vi "Pulsed BPSK Modulator - Channel 0.vi"() -> ()   [LabVIEW 2023]
uses:
  <vilib>/rvi/interface/nirviMethod/nirviMethod.xnode
  <vilib>/rvi/interface/nirviCloseFPGA/nirviCloseFPGA.xnode
  <vilib>/rvi/interface/nirviReadWriteControl/nirviReadWriteControl.xnode
  <vilib>/rvi/errors/niLvFpgaMergeErrorWithErrorCode.vi
  <vilib>/rvi/interface/Simulation/niFpgaSimulationCallBeginRW.vi
  <vilib>/rvi/errors/niLvFpgaAdjustHostInterfaceError.vi
  Support/Pulsed BPSK Host Support.lvlib
  <vilib>/addons/Modulation/niDMT.lvlib
  Shared/AWGN/AWGN.lvlib
  <vilib>/FPGAPlugInAG/Dynamic/niLvFpga_ReadFifo_Dynamic.vi
  <vilib>/addons/Modulation/Analog/controls/Complex Data Waveform.ctl
  <vilib>/addons/Modulation/niAMT.lvlib
  Shared/BER/Host/BER Host.lvclass
  Shared/FIR/FIR.lvlib
  Support/Public/FPGA Refnum.ctl
  Shared/AWGN/typedefs/Output Type Selection.ctl
  <vilib>/DLsc/v1/Host/Link Engine/DLsc Link Engine v1 Host.lvlib
  <vilib>/FPGAPlugInAG/Dynamic/niLvFpga_Close_Dynamic.vi
  2aa000c3-8f04-4506-bfc8-0c9442f73a61.vi
  5cab5cb4-fad3-4148-b0d2-6afb77881806.vi
  27528e13-72c1-4a4e-be7c-d3d202733046.vi
  35aca2bc-a3d1-4f8c-b8ac-3d3d75dd1f08.vi
  <vilib>/DLsc/v1/Host/Protocols/Aurora 64b66b/Extension/Aurora 64b66b Extension.lvlib
  <vilib>/DLsc/v1/Host/Link Engine/Disable Links - Single.vi
  <vilib>/addons/Modulation/Digital/General/MT Apply Matched Filter (Generic).vi
  <vilib>/addons/Modulation/Digital/General/MT Align to Ideal Symbols (Generic).vi
  <vilib>/Utility/error.llb/Error Cluster From Error Code.vi
  NiFpgaLv.dll
  <vilib>/DLsc/v1/Host/Link Engine/Enable Links - Single.vi
  <vilib>/DLsc/v1/Host/Link Engine/Commit Links - Single.vi
  <vilib>/DLsc/v1/Host/Protocols/Aurora 64b66b/Extension/Configure TX - Single.vi
  <vilib>/DLsc/v1/Host/Link Engine/Add Hardware - Single.vi
  <vilib>/FPGAPlugInAG/Dynamic/niLvFpga_Download_Dynamic.vi
  <vilib>/FPGAPlugInAG/Dynamic/niLvFpga_Run_Dynamic.vi
  <vilib>/DLsc/v1/Host/Link Engine/Close References - Single.vi
  <vilib>/FPGAPlugInAG/Dynamic/niLvFpga_ConfigureFifo_Dynamic.vi
  <vilib>/FPGAPlugInAG/Dynamic/niLvFpga_StartFifo_Dynamic.vi
  <vilib>/FPGAPlugInAG/Dynamic/niLvFpga_WriteFifo_Dynamic.vi
  <vilib>/userDefined/High Color/nirio_resource_hc.ctl
  Shared/BER/FPGA/PRBS/PRBS Degree Selection.ctl
  Shared/BER/FPGA/PRBS/PRBS.lvlib
panel:
  in  "disable DL":bool
  in  "enable DL":bool
  in  "Signal Parameters.0":T2={"Symbol Rate (Hz)"=400000000.0, "Pulse Parameters"={"Payload Length"=800, "Off Symbol Length"=800, "Preamble Symbol"=449838109, "PN Order"=4}} {"Pulse Parameters"."PN Order" items=["7", "9", "10", "11", "15", "17", "18", "20", "21", "22", "23", "25"]; "Pulse Parameters"."Preamble Symbol" format="%.0x"; "Symbol Rate (Hz)" format="%#_6p"}
  in  "Eb/N0 (dB).0":dbl=30.0 min=0.0 max=100.0 step=1.0 format="%.2g"
  in  "Power Scaling.0":dbl=1.0 min=0.0 max=1.0 step=0.002 format="%_5g"
  in  "Generation Mode.0":string(combo)="Pulsed BPSK Modulator"
  in  "Sweeping Type.0":enum16{"Eb/N0", "Power"}(ring)
  in  "Run Sweep":bool
  out "IQ Constellation":T3(graph)
  out "Bitfile Redownloaded":bool
  in  "Coprocessor Bitfile Path":path=path "C:/Users/ADG-RF/Desktop/Modems/pulsed_bpsk_modem_dmsc_7903_00_x420_single.lvbitx"
  in  "Coprocessor Device Name":T4="7903"
  in  "stop":bool
  out "Status":string
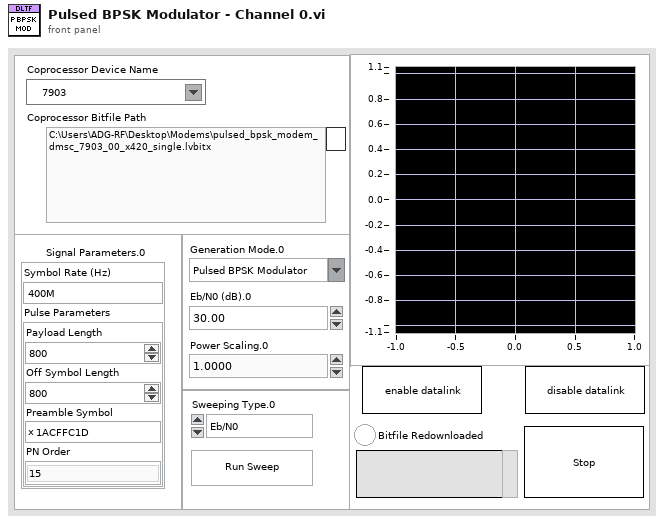
[diagram p1: front panel]
types:
  T1 = typedef "Modems Shared.lvlib/PRBS.lvlib/PRBS Degree Selection.ctl" = u16
  T2 = cluster{"Symbol Rate (Hz)":dbl, "Pulse Parameters":cluster{"Payload Length":u16, "Off Symbol Length":u16, "Preamble Symbol":i32, "PN Order":T1}}
  T3 = cluster{"constellation":dbl[], "oversampled data":dbl[]}[]
  T4 = typedef "nirio_resource_hc.ctl" = tag
  T5 = cluster{"dstepid":u16, "nummdata":fxp<+,5,5>, "pkttype":fxp<+,3,3>, "burst length":u16, "vector length":u16, "vc":fxp<+,6,6>}
  T6 = typedef "Pulsed BPSK Host Support.lvlib/FPGA Refnum.ctl" = refnum<k20>
  T7 = typedef "DLsc Link Engine v1 Host.lvlib/DLsc Session.lvclass/Session Handle.ctl" = refnum<data-value>
  T8 = typedef "DLsc Link Engine v1 Host.lvlib/DLsc Session.lvclass/Device Address Information.ctl" = cluster{"device name":string, "bitfile path":path}
  T9 = cluster{"On Symbol Count":u16, "Off Symbol Count":u16, "filter length":u16, "Preamble Count":u16}
  T10 = cluster{"AWGN Seed":fxp<+,25,25>, "AWGN scaling":fxp<+,16,0>, "output type selection":i16, "power scaling":fxp<+,16,0>}
  T11 = cluster{"filter select":enum8{"None", "I Inline", "I Cross", "Q Cross", "Q Inline"}, "coef load":bool, "coef write":bool, "coef data":fxp<+/-,18,1>}
  T12 = typedef "Modems Shared.lvlib/AWGN.lvlib/Output Type Selection.ctl" = enum16{"I16.1", "I16.2", "I16.3", "I16.4", "I16.5", "AWGN"}
  T13 = enum16{"FSK", "PSK", "QAM", "MSK", "PAM", "ASK", "CPM"}
  T14 = enum16{"none", "Raised Cosine", "Root Raised Cos", "Gaussian"}
  T15 = typedef "niAMT.lvlib/Complex Data Waveform.ctl" = cluster{"t0":dbl, "dt":dbl, "Y":cdb[]}
  T16 = cluster{"Inc":bool, "Sweeping Type":enum16{"Eb/N0", "Power"}, "Sweeping Start Point":cluster{"Eb/N0":dbl, "Power Scaling":dbl}, "Sweeping Current Point":cluster{"Eb/N0":dbl, "Power Scaling":dbl}}
  T17 = cluster{"Eb/N0 (dB).0":dbl, "Power Scaling.0":dbl}
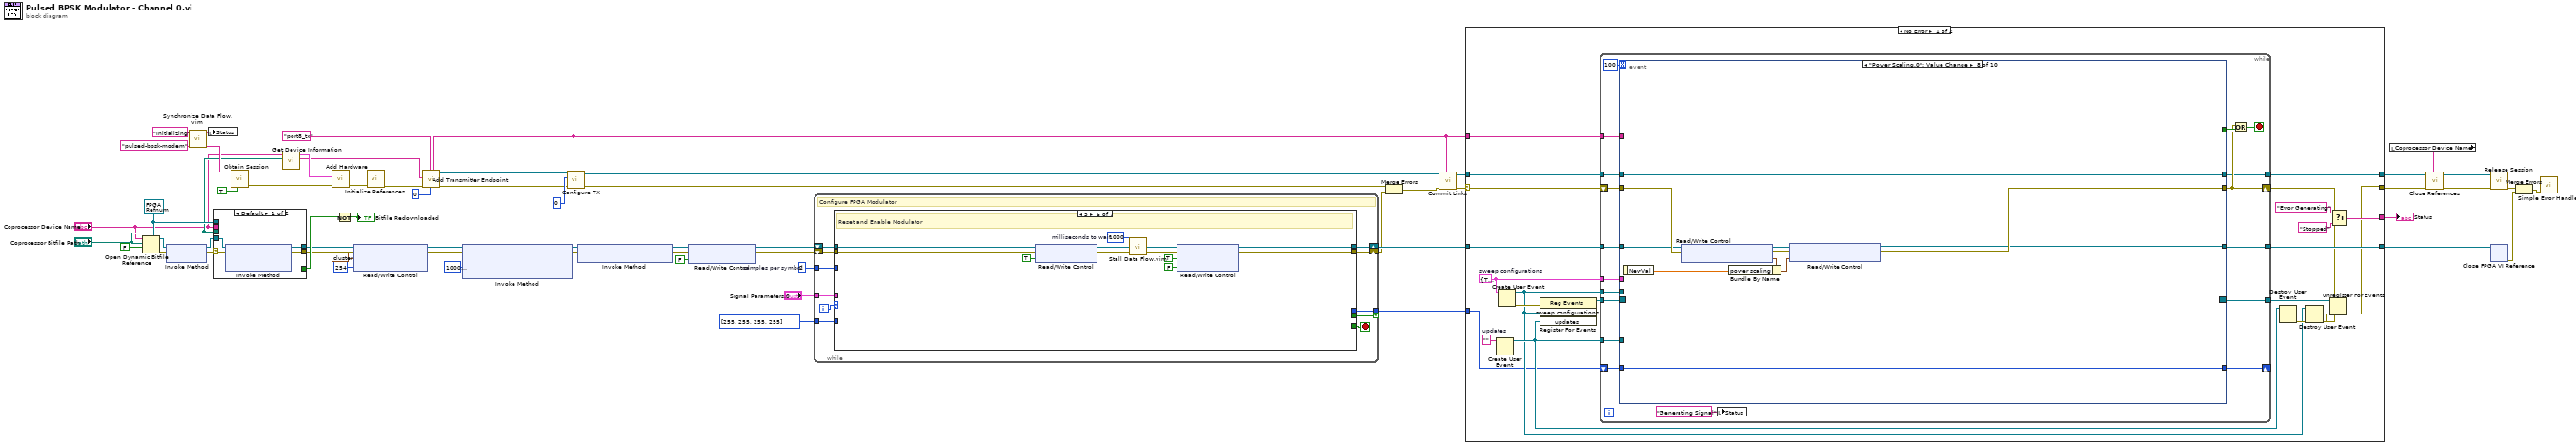
[diagram p0: block diagram]
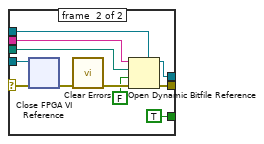
[diagram p2: hidden frame]
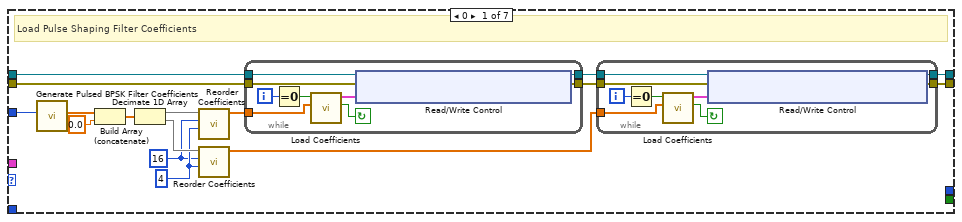
[diagram p3: hidden frame]
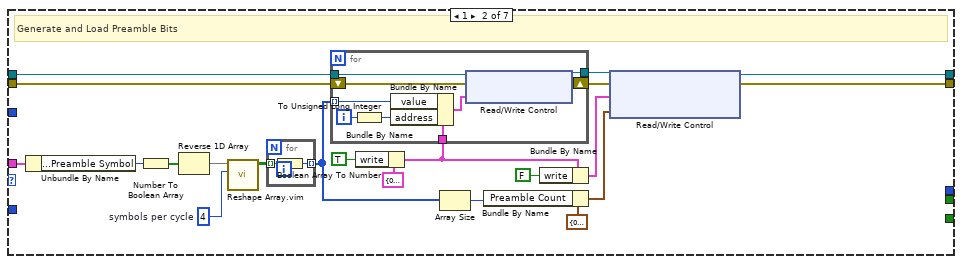
[diagram p4: hidden frame]
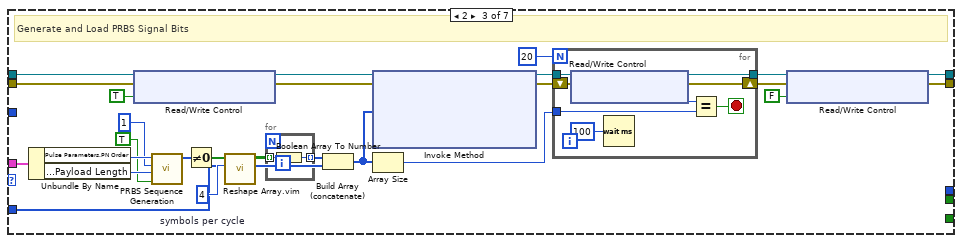
[diagram p5: hidden frame]
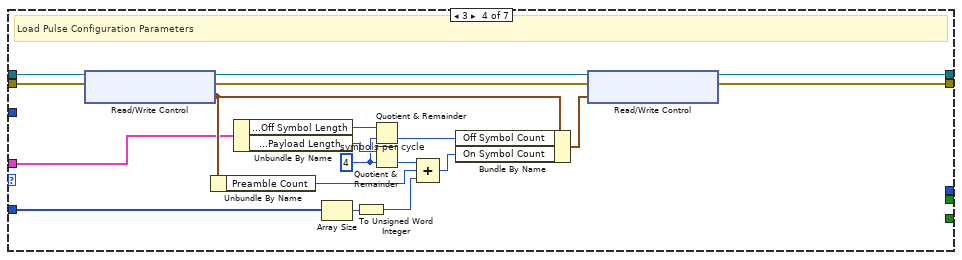
[diagram p6: hidden frame]
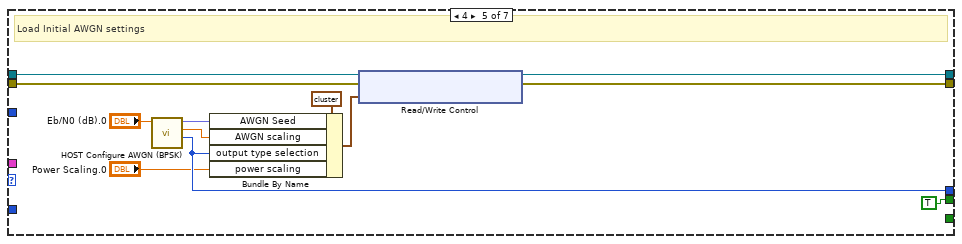
[diagram p7: hidden frame]
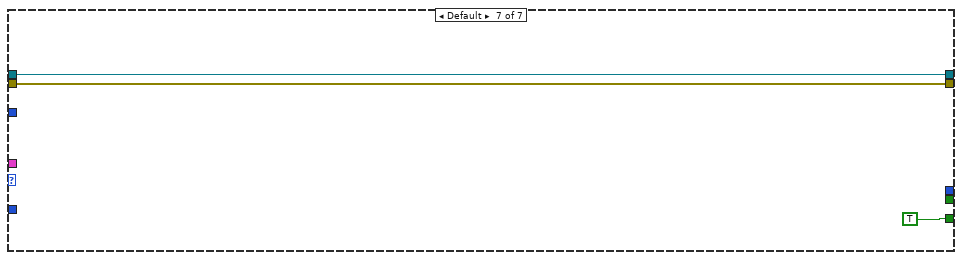
[diagram p8: hidden frame]
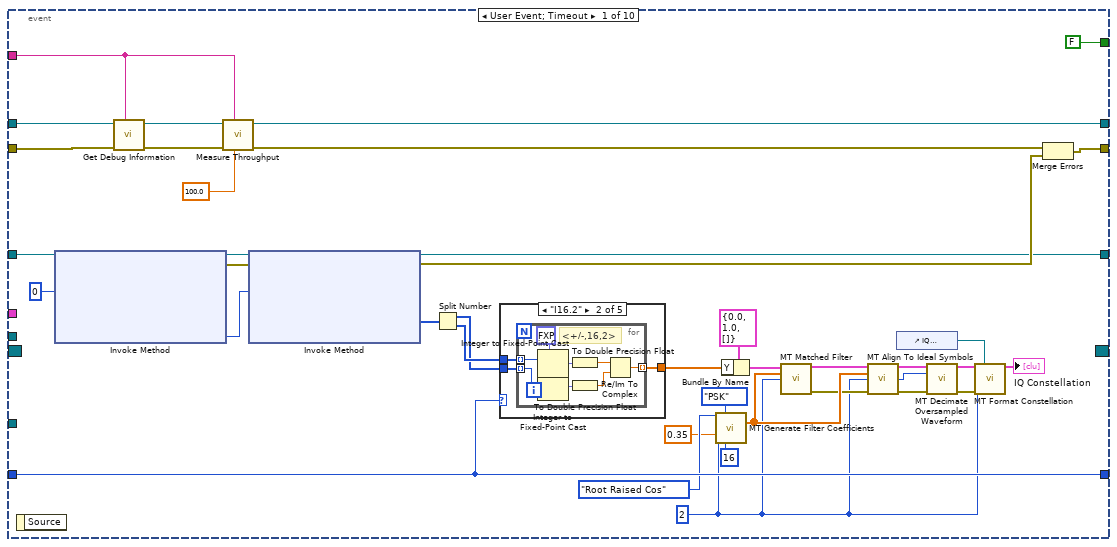
[diagram p9: hidden frame]
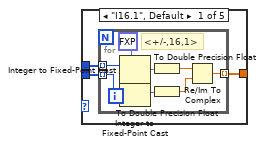
[diagram p10: hidden frame]
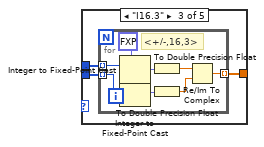
[diagram p11: hidden frame]
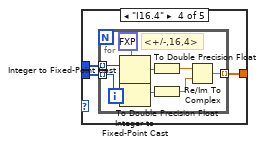
[diagram p12: hidden frame]
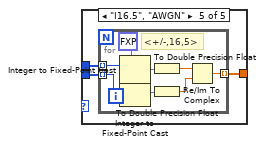
[diagram p13: hidden frame]
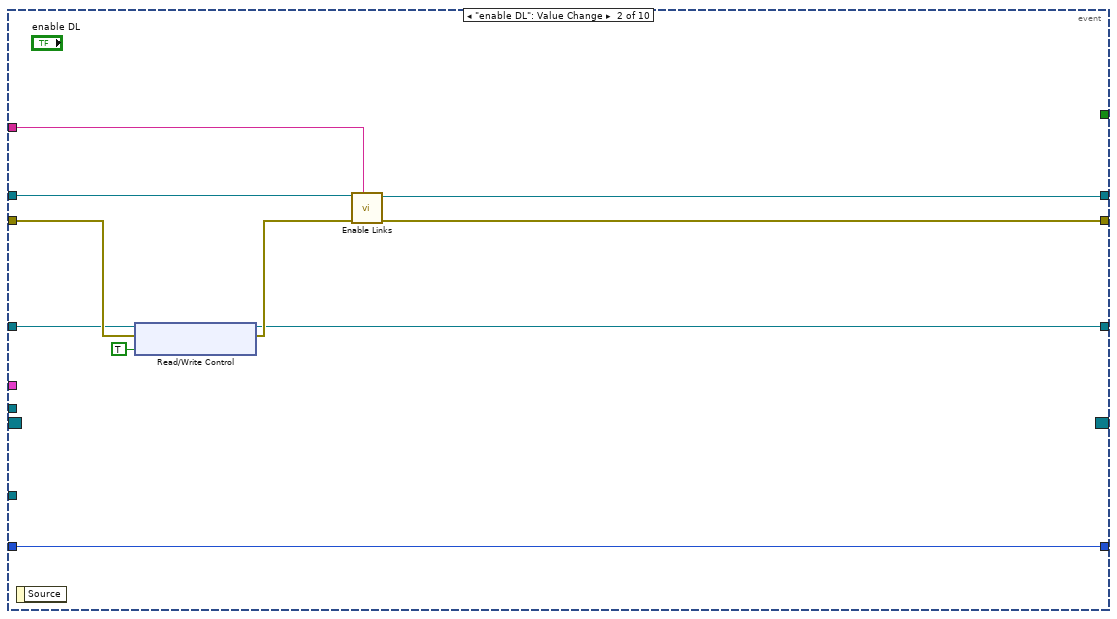
[diagram p14: hidden frame]
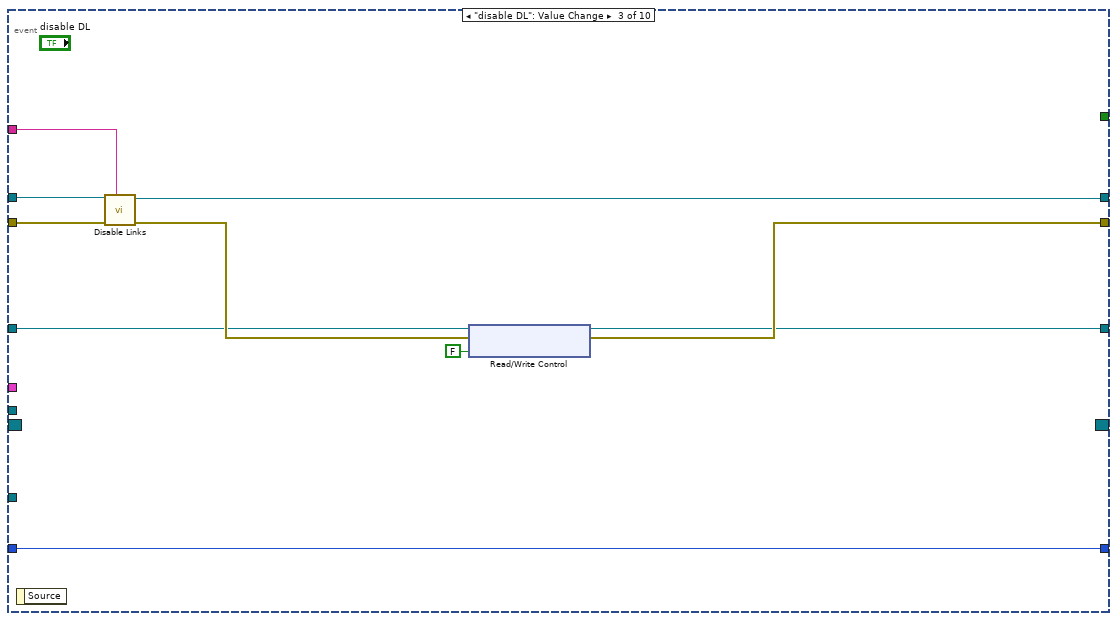
[diagram p15: hidden frame]
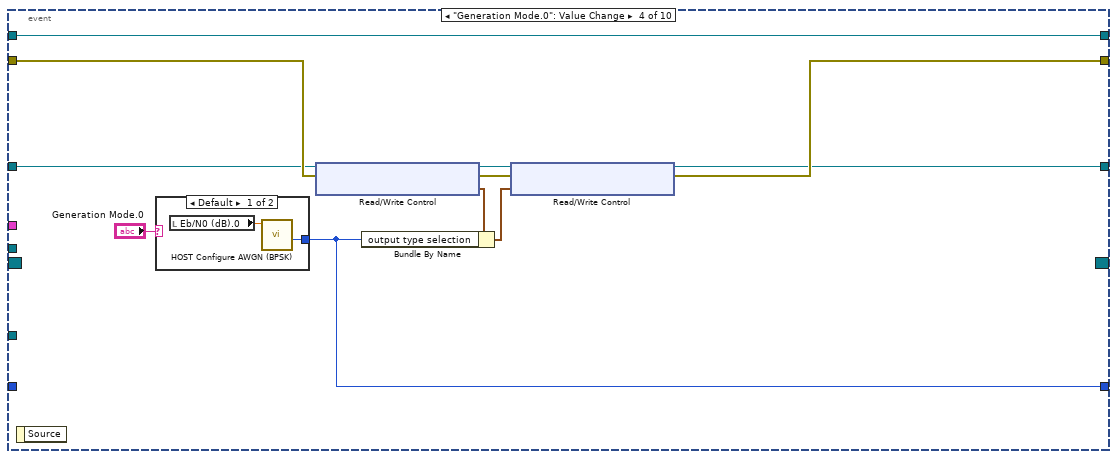
[diagram p16: hidden frame]
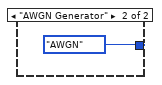
[diagram p17: hidden frame]
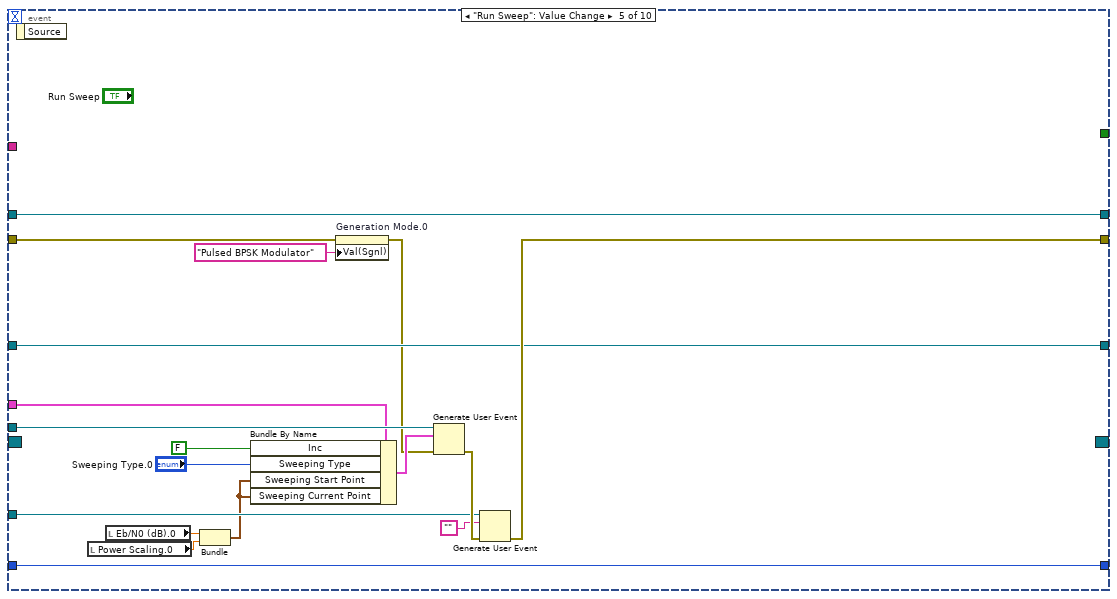
[diagram p18: hidden frame]
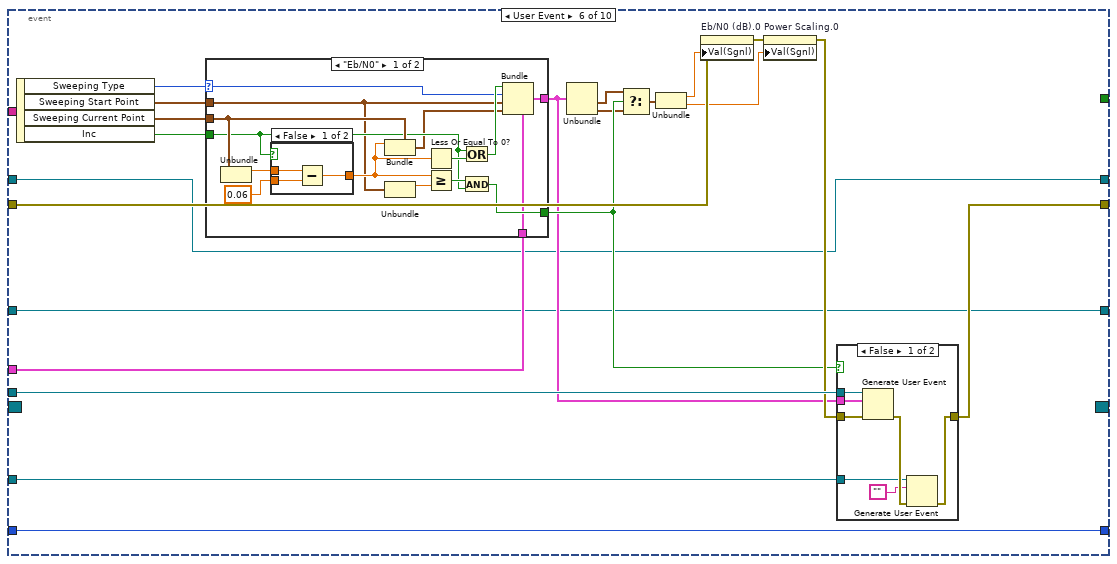
[diagram p19: hidden frame]
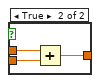
[diagram p20: hidden frame]
diagram:
  w36 = T6 refnum ("pulsed bpsk coprocessor refnum")
  w21 = 2  # samples per symbol
  n1 = Open Dynamic Bitfile Reference(0:"Coprocessor Device Name", 1:"Coprocessor Bitfile Path", 2:FALSE ("Run When Loaded"), 4:w36) -> (5:w63:T6, 8:w44:errorcluster)  [unwired: 1 in]
  n2 = xnode "Invoke Method"("FPGA VI Reference In"=w63, "error in"=w44) -> ("FPGA VI Reference Out"=w41:T6, "error out"=w40:errorcluster)
  n3 = call "Synchronize Data Flow.vim"("input 4"="pulsed-bpsk-modem", "input 1"="Initializing") -> ("output 4"=w25:string, "output 1"=w43:string)  [unwired: 2 in, 2 out]
  n4 = local write "Status"(w43) -> ()
  n5 = case shown="Default" w40 {
    selector: w40 -> [w66 w79]
    tunnel: [w68 w72] -> w31
    tunnel: [w67 w75] -> w30
    tunnel: w41 -> [w65 w77]
    tunnel: w36 -> [_ w73]
    tunnel: "Coprocessor Device Name" -> [_ w71]
    tunnel: "Coprocessor Bitfile Path" -> [_ w70]
    tunnel: [_ TRUE] -> w39
    frame #0 {
      n6 = xnode "Invoke Method"("FPGA VI Reference In"=w65, "error in"=w66) -> ("FPGA VI Reference Out"=w68:T6, "error out"=w67:errorcluster)  [unwired: 1 in]
    }
    frame #1 {
      n7 = xnode "Close FPGA VI Reference"("FPGA VI Reference In"=w77, "error in"=w79) -> ("error out"=w78:errorcluster)
      n8 = call <vilib>:"Clear Errors.vi"("error in (no error)"=w78) -> ("error out"=w76:errorcluster)  [unwired: 5 in, 1 out]
      n9 = Open Dynamic Bitfile Reference(0:w71, 1:w70, 2:FALSE ("Run When Loaded"), 3:w76, 4:w73) -> (5:w72:T6, 8:w75:errorcluster)
    }
  }
  n10 = call <vilib>:"Obtain Session.vi"("use remote engine (f)"=TRUE, "session name (\"\":default)"=w25) -> ("error out"=w27:errorcluster, "session out"=w28:T7)  [unwired: 6 in, 2 out]
  n11 = call <vilib>:"Get Device Information.vi"("bitfile path"="Coprocessor Bitfile Path", "device name"="Coprocessor Device Name") -> ("device name out"=w26:string, "device address information"=w54:T8)  [unwired: 7 in, 1 out]
  n12 = call-poly <vilib>:"Add Hardware.vi"("error in"=w27, "device"=w54, "session in"=w28) -> ("error out"=w5:errorcluster, "session out"=w6:T7)  [unwired: 7 in]
  n13 = Not(x=w39) -> (.not. x?=→"Bitfile Redownloaded":bool)
  n14 = xnode "Read/Write Control"("FPGA VI Reference In"=w31, "error in"=w30, "header parameters.0"=T5 {"dstepid"=0, "nummdata"=0.0, "pkttype"=6.0, "burst length"=506, "vector length"=1012, "vc"=1.0} ("header parameters"), "aurora frame length.0"=u16 254 ("packet length")) -> ("FPGA VI Reference Out"=w11:T6, "error out"=w10:errorcluster)
  n15 = call <vilib>:"Initialize References.vi"("error in"=w5, "session in"=w6) -> ("error out"=w3:errorcluster, "session out"=w4:T7)  [unwired: 8 in]
  n16 = call <vilib>:"Add Transmitter Endpoint.vi"("transmitter instance (0)"=u8 0, "link name"="port8_tx", "error in"=w3, "transmitter device name"=w26, "session in"=w4) -> ("error out"=w1:errorcluster, "session out"=w2:T7, "link name out"=w22:string)  [unwired: 2 in, 2 out]
  n17 = xnode "Invoke Method"("FPGA VI Reference In"=w11, "error in"=w10, "Requested Depth"=u32 10000000) -> ("FPGA VI Reference Out"=w62:T6, "error out"=w61:errorcluster)  [unwired: 1 out]
  n18 = call-poly <vilib>:"Configure TX.vi"("link name (\"\":default)"=w22, "error in"=w1, "frame size"=u16 0 ("tx frame size"), "session in"=w2) -> ("error out"=w17:errorcluster, "session out"=w8:T7)  [unwired: 6 in]
  n19 = xnode "Invoke Method"("FPGA VI Reference In"=w62, "error in"=w61) -> ("FPGA VI Reference Out"=w35:T6, "error out"=w34:errorcluster)
  n20 = xnode "Read/Write Control"("FPGA VI Reference In"=w35, "error in"=w34, "enable modulator.0"=FALSE ("enable modulator")) -> ("FPGA VI Reference Out"=w33:T6, "error out"=w32:errorcluster)
  n21 = while {
    tunnel: "Signal Parameters.0" -> [w88]
    shift-right: [w87] -> w48
    shift-left: w33 -> [w90]
    shift-right: [w86] -> w47
    shift-left: w32 -> [w89]
    tunnel: u8[] [255, 255, 255, 255] ("array") -> [w83]
    tunnel: [w82] -> w45 if=w81
    tunnel: w21 -> [w80]
    i -> [w84]
    stop <- w85 stop-if-true
    # "Configure FPGA Modulator"
    n22 = case shown="5" w84 {
      tunnel: w90 -> [w97 w140 w162 w201 w223 w228 w236]
      tunnel: w89 -> [w96 w139 w161 w200 w222 w227 w235]
      tunnel: w88 -> [_ w127 w158 w193 _ _ _]
      tunnel: [w93 w133 w160 w195 w217 w226 w236] -> w87
      tunnel: [w92 w132 w159 w202 w216 w225 w235] -> w86
      tunnel: [_ _ _ _ _ _ TRUE] -> w85
      tunnel: w83 -> [_ _ w157 w194 _ _ _]
      tunnel: [_ _ _ _ w215 _ _] -> w82
      tunnel: [_ _ _ _ TRUE _ _] -> w81
      tunnel: w80 -> [w91 _ _ _ _ _ _]
      frame 0 {
        w99 = 4 ("spc")
        w98 = 16 ("num taps")
        # "Load Pulse Shaping Filter Coefficients"
        n23 = call "Generate Pulsed BPSK Filter Coefficients.vi"("samples per symbol"=w91) -> ("pulse shaping filter coefficients"=w106:dbl[])  [unwired: 7 in, 3 out]
        n24 = Build Array (concatenate)(w106, 0.0) -> (w105:dbl[])
        n25 = Decimate 1D Array(w105) -> (w104:dbl[], w102:dbl[])
        n26 = call "Reorder Coefficients.vi"("spc"=w99, "num taps"=w98, "taps"=w104) -> ("reordered taps"=w103:dbl[])  [unwired: 8 in]
        n27 = call "Reorder Coefficients.vi"("spc"=w99, "num taps"=w98, "taps"=w102) -> ("reordered taps"=w101:dbl[])  [unwired: 8 in]
        n28 = while {
          tunnel: w97 -> [w123]
          tunnel: w96 -> [w122]
          tunnel: w103 -> [w124]
          tunnel: [w119] -> w95
          tunnel: [w118] -> w94
          i -> [w117]
          stop <- w120 continue-if-true
          n29 = Equal To 0?(x=w117) -> (x = 0?=w116:bool)
          n30 = call "Load Coefficients.vi"("coefficients"=w124, "load"=w116) -> ("loading"=w120:bool, "filter coefficients"=w121:T11)  [unwired: 8 in]
          n31 = xnode "Read/Write Control"("FPGA VI Reference In"=w123, "error in"=w122, "pulse shaping filter coefficients odd.0"=w121) -> ("FPGA VI Reference Out"=w119:T6, "error out"=w118:errorcluster)
        }
        n32 = while {
          tunnel: w95 -> [w114]
          tunnel: w94 -> [w113]
          tunnel: w101 -> [w115]
          tunnel: [w110] -> w92
          tunnel: [w107] -> w93
          i -> [w109]
          stop <- w111 continue-if-true
          n33 = Equal To 0?(x=w109) -> (x = 0?=w108:bool)
          n34 = call "Load Coefficients.vi"("coefficients"=w115, "load"=w108) -> ("loading"=w111:bool, "filter coefficients"=w112:T11)  [unwired: 8 in]
          n35 = xnode "Read/Write Control"("FPGA VI Reference In"=w114, "error in"=w113, "pulse shaping filter coefficients even.0"=w112) -> ("FPGA VI Reference Out"=w107:T6, "error out"=w110:errorcluster)
        }
      }
      frame 1 {
        w125 = 4  # symbols per cycle
        # "Generate and Load Preamble Bits"
        n36 = Unbundle By Name(w127) -> ("Pulse Parameters.Preamble Symbol"=w145:i32)
        n37 = Number To Boolean Array(number=w145) -> (Boolean array=w143:bool[])
        n38 = Reverse 1D Array(array=w143) -> (reversed array=w126:bool[])
        n39 = call "Reshape Array.vim"("column size"=w125, "input array"=w126) -> ("output array"=w144:bool[][])  [unwired: 9 in]
        n40 = for {
          tunnel: w144 -> [w156] mode=indexing
          tunnel: [w155] -> w129 mode=indexing
          n41 = Boolean Array To Number(Boolean array=w156) -> (number=w155:u8)
        }
        n42 = Bundle By Name(cluster=cluster{"address":u32, "write":bool, "value":u8} {"address"=0, "write"=TRUE, "value"=0} ("preamble write"), "write"=TRUE) -> (w134:cluster{"address":u32, "write":bool, "value":u8})
        n43 = for {
          tunnel: w140 -> [w154]
          tunnel: [w152] -> w142
          shift-right: [w151] -> w141
          shift-left: w139 -> [w153]
          tunnel: w129 -> [w150] mode=indexing
          tunnel: w134 -> [w146]
          i -> [w149]
          n44 = To Unsigned Long Integer(number=w149) -> (unsigned 32bit integer=w148:u32)
          n45 = Bundle By Name(cluster=w146, "value"=w150, "address"=w148) -> (w147:cluster{"address":u32, "write":bool, "value":u8})
          n46 = xnode "Read/Write Control"("FPGA VI Reference In"=w154, "error in"=w153, "preamble write.0"=w147) -> ("FPGA VI Reference Out"=w152:T6, "error out"=w151:errorcluster)
        }
        n47 = Array Size(array=w129) -> (size(s)=w130:i32)
        n48 = Bundle By Name(cluster=T9 {"On Symbol Count"=0, "Off Symbol Count"=0, "filter length"=0, "Preamble Count"=0} ("pulse configuration"), "Preamble Count"=w130) -> (w128:T9)
        n49 = Bundle By Name(cluster=w134, "write"=FALSE) -> (w135:cluster{"address":u32, "write":bool, "value":u8})
        n50 = xnode "Read/Write Control"("FPGA VI Reference In"=w142, "error in"=w141, "preamble write.0"=w135, "pulse configuration.0"=w128) -> ("FPGA VI Reference Out"=w133:T6, "error out"=w132:errorcluster)
      }
      frame 2 {
        w180 = 4  # symbols per cycle
        # "Generate and Load PRBS Signal Bits"
        n51 = Unbundle By Name(w158) -> ("Pulse Parameters.PN Order"=w176:T1, "Pulse Parameters.Payload Length"=w177:u16)
        n52 = xnode "Read/Write Control"("FPGA VI Reference In"=w162, "error in"=w161, "update bit generation.0"=TRUE ("update bit generation")) -> ("FPGA VI Reference Out"=w169:T6, "error out"=w173:errorcluster)
        n53 = call "PRBS Sequence Generation.vi"("backward"=TRUE, "total bits"=w177, "seed"=u32 1, "PRBS degree"=w176) -> ("bit stream"=w178:i16[])  [unwired: 6 in, 1 out]
        n54 = Not Equal To 0?(x=w178) -> (x != 0?=w181:bool[])
        n55 = call "Reshape Array.vim"("column size"=w180, "input array"=w181) -> ("output array"=w179:bool[][])  [unwired: 9 in]
        n56 = for {
          tunnel: w179 -> [w192] mode=indexing
          tunnel: [w191] -> w182 mode=indexing
          n57 = Boolean Array To Number(Boolean array=w192) -> (number=w191:u8)
        }
        n58 = Build Array (concatenate)(w182, w157) -> (w163:u8[])
        n59 = xnode "Invoke Method"("FPGA VI Reference In"=w169, "error in"=w173, "Data"=w163) -> ("FPGA VI Reference Out"=w172:T6, "error out"=w171:errorcluster)  [unwired: 1 in, 1 out]
        n60 = Array Size(array=w163) -> (size(s)=w170:i32)
        n61 = for {
          N: 20 -> [_]
          tunnel: w172 -> [w190]
          tunnel: w170 -> [w187]
          tunnel: [w184] -> w168
          shift-right: [w183] -> w167
          shift-left: w171 -> [w189]
          stop <- w186 stop-if-true
          n62 = xnode "Read/Write Control"("FPGA VI Reference In"=w190, "error in"=w189) -> ("FPGA VI Reference Out"=w184:T6, "error out"=w183:errorcluster, "bit stream length.0"=w188:u32)
          n63 = Wait (ms)(milliseconds to wait=u32 100) -> ()  [unwired: 1 out]
          n64 = Equal?(x=w188, y=w187) -> (x = y?=w186:bool)
        }
        n65 = xnode "Read/Write Control"("FPGA VI Reference In"=w168, "error in"=w167, "update bit generation.0"=FALSE ("update bit generation")) -> ("FPGA VI Reference Out"=w160:T6, "error out"=w159:errorcluster)
      }
      frame 3 {
        w209 = u16 4  # symbols per cycle
        # "Load Pulse Configuration Parameters"
        n66 = xnode "Read/Write Control"("FPGA VI Reference In"=w201, "error in"=w200) -> ("FPGA VI Reference Out"=w199:T6, "error out"=w198:errorcluster, "pulse configuration.0"=w197:T9)
        n67 = Unbundle By Name(w197) -> ("Preamble Count"=w196:u16)
        n68 = Unbundle By Name(w193) -> ("Pulse Parameters.Off Symbol Length"=w211:u16, "Pulse Parameters.Payload Length"=w210:u16)
        n69 = Array Size(array=w194) -> (size(s)=w207:i32)
        n70 = To Unsigned Word Integer(number=w207) -> (unsigned 16bit integer=w204:u16)
        n71 = Quotient & Remainder(x=w211, y=w209) -> (floor(x/y)=w206:u16)  [unwired: 1 out]
        n72 = Quotient & Remainder(x=w210, y=w209) -> (floor(x/y)=w205:u16)  [unwired: 1 out]
        n73 = Compound Arithmetic op=ADD(w205, w196, w204) -> (w203:u16)
        n74 = Bundle By Name(cluster=w197, "Off Symbol Count"=w206, "On Symbol Count"=w203) -> (w208:T9)
        n75 = xnode "Read/Write Control"("FPGA VI Reference In"=w199, "error in"=w198, "pulse configuration.0"=w208) -> ("FPGA VI Reference Out"=w195:T6, "error out"=w202:errorcluster)
      }
      frame 4 {
        # "Load Initial AWGN settings"
        n76 = call "HOST Configure AWGN (BPSK).vi"("E0/Nb"="Eb/N0 (dB).0") -> ("output data type"=w215:T12, "noise std deviation\n(unity signal power)"=w221:dbl, "seed"=w220:fxp<+,25,25>)  [unwired: 8 in]
        n77 = Bundle By Name(cluster=T10 {"AWGN Seed"=0.0, "AWGN scaling"=0.0, "output type selection"=0, "power scaling"=0.0} ("modulator configurations"), "AWGN Seed"=w220, "AWGN scaling"=w221, "output type selection"=w215, "power scaling"="Power Scaling.0") -> (w218:T10)
        n78 = xnode "Read/Write Control"("FPGA VI Reference In"=w223, "error in"=w222, "modulator configurations.0"=w218) -> ("FPGA VI Reference Out"=w217:T6, "error out"=w216:errorcluster)
      }
      frame 5 {
        w224 = u32 1000  # milliseconds to wait
        # "Reset and Enable Modulator"
        n79 = xnode "Read/Write Control"("FPGA VI Reference In"=w228, "error in"=w227, "reset modulator.0"=TRUE ("reset modulator")) -> ("FPGA VI Reference Out"=w231:T6, "error out"=w232:errorcluster)
        n80 = call "Stall Data Flow.vim"("value in"=w231, "milliseconds to wait"=w224) -> ("value out"=w234:T6)  [unwired: 1 out]
        n81 = xnode "Read/Write Control"("FPGA VI Reference In"=w234, "error in"=w232, "reset modulator.0"=TRUE ("reset modulator"), "reset modulator.0"=FALSE ("enable modulator")) -> ("FPGA VI Reference Out"=w226:T6, "error out"=w225:errorcluster)
      }
      frame Default {
      }
    }
  }
  n82 = Merge Errors(w17, w47) -> (w7:errorcluster)
  n83 = call-poly <vilib>:"Commit Links.vi"("link name (\"\":all)"=w22, "error in"=w7, "session in"=w8) -> ("error out"=w15:errorcluster, "session out"=w16:T7)  [unwired: 7 in]
  n84 = case shown="No Error" w15 {
    selector: w15 -> [w240 w530]
    tunnel: w16 -> [w241 w531]
    tunnel: w22 -> [w242 _]
    tunnel: [w239 w531] -> w51
    tunnel: [w238 w530] -> w50
    tunnel: [w258 w528] -> w59
    tunnel: [w255 "Link Failed to Initialize" ("t")] -> w64
    tunnel: w48 -> [w245 w528]
    tunnel: w45 -> [w244 _]
    frame No Error {
      w243 = T16 {"Inc"=TRUE, "Sweeping Type"=enum."Power", "Sweeping Start Point"={"Eb/N0"=0.0, "Power Scaling"=0.0}, "Sweeping Current Point"={"Eb/N0"=0.0, "Power Scaling"=0.0}}  # sweep configurations
      w252 = ""  # updates
      n85 = Create User Event(user event datatype=w252) -> (user event=w247:refnum<user-event>)  [unwired: 1 in, 1 out]
      n86 = Create User Event(user event datatype=w243) -> (user event=w246:refnum<user-event>, error out=w254:errorcluster)  [unwired: 1 in]
      n87 = register-events(error in=w254, w246, w247) -> (reference out=w253:refnum<event-registration>)  [unwired: 1 in, 1 out]
      n88 = while {
        shift-right: [w271] -> w250
        shift-left: w240 -> [w276]
        shift-right: [w268] -> _
        shift-left: w244 -> [w269]
        tunnel: w241 -> [w270]
        tunnel: [w267] -> w258
        tunnel: [w266] -> w239
        tunnel: w242 -> [w265]
        tunnel: w253 -> [w264]
        tunnel: w246 -> [w263]
        tunnel: w247 -> [w262]
        tunnel: [w261] -> w251
        tunnel: w245 -> [w260]
        tunnel: w243 -> [w259]
        stop <- w272 stop-if-true
        n89 = event shown="[7] \"Power Scaling.0\": Value Change" {
          selector: w264 -> [_ _ _ _ _ _ _ _ _ _]
          dyn-events: [_ _ _ _ _ _ _ _ _ _] -> w261
          timeout: 100 ("milliseconds to wait") -> [_ _ _ _ _ _ _ _ _ _]
          tunnel: w276 -> [w278 w373 w388 w397 w404 w437 w502 w516 w522 w526]
          tunnel: [FALSE ("done?") _ _ _ _ _ _ _ w519 TRUE ("done?")] -> w275
          tunnel: [w287 w376 w382 w400 w413 w439 w505 w512 w522 w526] -> w271
          tunnel: w269 -> [w299 w375 w385 _ w421 w442 _ w517 w521 w525]
          tunnel: [w299 w375 w385 w391 w421 w442 w496 w517 w521 w525] -> w268
          tunnel: w270 -> [w281 w379 w389 w398 w420 w422 w503 w515 w520 w524]
          tunnel: [w288 w370 w380 w399 w407 w423 w504 w511 w518 w523] -> w267
          tunnel: [w279 w378 w387 w398 w420 w422 w503 w515 w520 w524] -> w266
          tunnel: w265 -> [w282 w377 w386 _ _ _ _ _ _ _]
          tunnel: w263 -> [_ _ _ _ w419 w440 _ _ _ _]
          tunnel: w262 -> [_ _ _ _ w417 w438 _ _ _ _]
          tunnel: w259 -> [_ _ _ _ w412 w435 _ _ _ _]
          tunnel: w260 -> [w290 w371 w381 w390 w407 w423 w493 w508 w518 w523]
          event User Event; Timeout {
            w289 = 2
            n90 = event-data() -> ()  [unwired: 1 in, 1 out]
            n91 = xnode "Invoke Method"("FPGA VI Reference In"=w290, "Number of Elements"=u32 0) -> ("FPGA VI Reference Out"=w311:T6, "error out"=w310:errorcluster, "Elements Remaining"=w307:u32)  [unwired: 2 in, 1 out]
            n92 = call <vilib>:"Get Debug Information.vi"("link name"=w282, "error in"=w278, "session in"=w281) -> ("error out"=w284:errorcluster, "session out"=w283:T7)  [unwired: 5 in, 2 out]
            n93 = call <vilib>:"Measure Throughput.vi"("measurement interval (500ms)"=100.0 ("thruput meas time (ms)"), "link name"=w282, "error in"=w284, "session in"=w283) -> ("error out"=w280:errorcluster, "session out"=w279:T7)  [unwired: 4 in, 2 out]
            n94 = xnode "Invoke Method"("FPGA VI Reference In"=w311, "error in"=w310, "Number of Elements"=w307) -> ("FPGA VI Reference Out"=w288:T6, "error out"=w304:errorcluster, "Data"=w277:u32[])  [unwired: 1 in, 1 out]
            n95 = Split Number(x=w277) -> (hi(x)=w305:u16[], lo(x)=w306:u16[])
            n96 = case shown="\"I16.2\"" w299 {
              tunnel: [w317 w328 w339 w350 w361] -> w314
              tunnel: w306 -> [w316 w327 w338 w349 w360]
              tunnel: w305 -> [w315 w326 w337 w348 w359]
              frame "I16.1", Default {
                n97 = for {
                  tunnel: w316 -> [w325] mode=indexing
                  tunnel: w315 -> [w324] mode=indexing
                  tunnel: [w321] -> w317 mode=indexing
                  w320 = fxp<+/-,16,1> 0.0 ("fixed-point type")
                  # "<+/-,16,1>"
                  n98 = Integer to Fixed-Point Cast(fixed-point type=w320, integer=w325) -> (fixed-point=w323:fxp<+/-,16,1>)
                  n99 = Integer to Fixed-Point Cast(fixed-point type=w320, integer=w324) -> (fixed-point=w322:fxp<+/-,16,1>)
                  n100 = To Double Precision Float(number=w323) -> (double precision float=w318:dbl)
                  n101 = To Double Precision Float(number=w322) -> (double precision float=w319:dbl)
                  n102 = Re/Im To Complex(1:w319, 2:w318) -> (0:w321:cdb)
                }
              }
              frame "I16.2" {
                n103 = for {
                  tunnel: w327 -> [w336] mode=indexing
                  tunnel: w326 -> [w335] mode=indexing
                  tunnel: [w332] -> w328 mode=indexing
                  w331 = fxp<+/-,16,2> 0.0 ("fixed-point type")
                  # "<+/-,16,2>"
                  n104 = Integer to Fixed-Point Cast(fixed-point type=w331, integer=w336) -> (fixed-point=w334:fxp<+/-,16,2>)
                  n105 = Integer to Fixed-Point Cast(fixed-point type=w331, integer=w335) -> (fixed-point=w333:fxp<+/-,16,2>)
                  n106 = To Double Precision Float(number=w334) -> (double precision float=w329:dbl)
                  n107 = To Double Precision Float(number=w333) -> (double precision float=w330:dbl)
                  n108 = Re/Im To Complex(1:w330, 2:w329) -> (0:w332:cdb)
                }
              }
              frame "I16.3" {
                n109 = for {
                  tunnel: w338 -> [w347] mode=indexing
                  tunnel: w337 -> [w346] mode=indexing
                  tunnel: [w343] -> w339 mode=indexing
                  w342 = fxp<+/-,16,3> 0.0 ("fixed-point type")
                  # "<+/-,16,3>"
                  n110 = Integer to Fixed-Point Cast(fixed-point type=w342, integer=w347) -> (fixed-point=w345:fxp<+/-,16,3>)
                  n111 = Integer to Fixed-Point Cast(fixed-point type=w342, integer=w346) -> (fixed-point=w344:fxp<+/-,16,3>)
                  n112 = To Double Precision Float(number=w345) -> (double precision float=w340:dbl)
                  n113 = To Double Precision Float(number=w344) -> (double precision float=w341:dbl)
                  n114 = Re/Im To Complex(1:w341, 2:w340) -> (0:w343:cdb)
                }
              }
              frame "I16.4" {
                n115 = for {
                  tunnel: w349 -> [w358] mode=indexing
                  tunnel: w348 -> [w357] mode=indexing
                  tunnel: [w354] -> w350 mode=indexing
                  w353 = fxp<+/-,16,4> 0.0 ("fixed-point type")
                  # "<+/-,16,4>"
                  n116 = Integer to Fixed-Point Cast(fixed-point type=w353, integer=w358) -> (fixed-point=w356:fxp<+/-,16,4>)
                  n117 = Integer to Fixed-Point Cast(fixed-point type=w353, integer=w357) -> (fixed-point=w355:fxp<+/-,16,4>)
                  n118 = To Double Precision Float(number=w356) -> (double precision float=w351:dbl)
                  n119 = To Double Precision Float(number=w355) -> (double precision float=w352:dbl)
                  n120 = Re/Im To Complex(1:w352, 2:w351) -> (0:w354:cdb)
                }
              }
              frame "I16.5", "AWGN" {
                n121 = for {
                  tunnel: w360 -> [w369] mode=indexing
                  tunnel: w359 -> [w368] mode=indexing
                  tunnel: [w365] -> w361 mode=indexing
                  w364 = fxp<+/-,16,5> 0.0 ("fixed-point type")
                  # "<+/-,16,5>"
                  n122 = Integer to Fixed-Point Cast(fixed-point type=w364, integer=w369) -> (fixed-point=w367:fxp<+/-,16,5>)
                  n123 = Integer to Fixed-Point Cast(fixed-point type=w364, integer=w368) -> (fixed-point=w366:fxp<+/-,16,5>)
                  n124 = To Double Precision Float(number=w367) -> (double precision float=w362:dbl)
                  n125 = To Double Precision Float(number=w366) -> (double precision float=w363:dbl)
                  n126 = Re/Im To Complex(1:w363, 2:w362) -> (0:w365:cdb)
                }
              }
            }
            n127 = call <vilib>:"MT Generate Filter Coefficients.vi"("pulse shaping filter (none)"=T14."Root Raised Cos", "modulation type"=T13."PSK", "pulse shaping samples per symbol (16)"=w289, "matched samples per symbol (16)"=w289, "filter parameter"=0.35, "filter length (symbols)"=16) -> ("matched filter coefficients"=w293:dbl[])  [unwired: 7 in, 2 out]
            n128 = Bundle By Name(cluster=T15 {"t0"=0.0, "dt"=1.0, "Y"=[]} ("waveform"), "Y"=w314) -> (w298:T15)
            n129 = call-poly <vilib>:"MT Matched Filter.vi"("input complex waveform"=w298, "matched filter coefficients"=w293, "samples per symbol (16)"=w289) -> ("output complex waveform"=w297:T15, "error out"=w291:errorcluster)  [unwired: 11 in]
            n130 = call-poly <vilib>:"MT Align To Ideal Symbols.vi"("input complex waveform"=w297, "matched filter coefficients"=w293, "samples per symbol (16)"=w289, "error in (no error)"=w291) -> ("output complex waveform"=w303:T15, "error out"=w302:errorcluster)  [unwired: 9 in, 1 out]
            n131 = control-ref of="IQ Constellation"() -> (w312:refnum<vi>)
            n132 = call <vilib>:"MT Decimate Oversampled Waveform.vi"("input complex waveform"=w303, "decimation factor"=w289, "error in (no error)"=w302) -> ("output complex waveform"=w301:T15, "error out"=w300:errorcluster)  [unwired: 11 in]
            n133 = call <vilib>:"MT Format Constellation.vi"("waveform"=w301, "constellation reference"=w312, "samples per symbol"=w289, "error in (no error)"=w300) -> ("constellation graph"=→"IQ Constellation":T3)  [unwired: 10 in, 1 out]
            n134 = Merge Errors(w280, w304) -> (w287:errorcluster)
          }
          event "enable DL": Value Change {
            n135 = event-data() -> ()  [unwired: 1 in, 1 out]
            n136 = xnode "Read/Write Control"("FPGA VI Reference In"=w371, "error in"=w373, "enable modulator.0"=TRUE ("enable modulator")) -> ("FPGA VI Reference Out"=w370:T6, "error out"=w372:errorcluster)
            n137 = call-poly <vilib>:"Enable Links.vi"("link name (\"\":all)"=w377, "error in"=w372, "session in"=w379) -> ("error out"=w376:errorcluster, "session out"=w378:T7)  [unwired: 7 in]
          }
          event "disable DL": Value Change {
            n138 = event-data() -> ()  [unwired: 1 in, 1 out]
            n139 = call-poly <vilib>:"Disable Links.vi"("link name (\"\":all)"=w386, "error in"=w388, "session in"=w389) -> ("error out"=w383:errorcluster, "session out"=w387:T7)  [unwired: 7 in]
            n140 = xnode "Read/Write Control"("FPGA VI Reference In"=w381, "error in"=w383, "enable modulator.0"=FALSE ("enable modulator")) -> ("FPGA VI Reference Out"=w380:T6, "error out"=w382:errorcluster)
          }
          event "Generation Mode.0": Value Change {
            n141 = event-data() -> ()  [unwired: 1 in, 1 out]
            n142 = case shown="Default" "Generation Mode.0" {
              tunnel: [w401 Output_Type_Selection."AWGN" ("output data type")] -> w391
              frame Default {
                n143 = local read "Eb/N0 (dB).0"() -> (w402:dbl)
                n144 = call "HOST Configure AWGN (BPSK).vi"("E0/Nb"=w402) -> ("output data type"=w401:T12)  [unwired: 8 in, 2 out]
              }
              frame "AWGN Generator" {
              }
            }
            n145 = xnode "Read/Write Control"("FPGA VI Reference In"=w390, "error in"=w397) -> ("FPGA VI Reference Out"=w396:T6, "error out"=w395:errorcluster, "modulator configurations.0"=w394:T10)
            n146 = Bundle By Name(cluster=w394, "output type selection"=w391) -> (w393:T10)
            n147 = xnode "Read/Write Control"("FPGA VI Reference In"=w396, "error in"=w395, "modulator configurations.0"=w393) -> ("FPGA VI Reference Out"=w399:T6, "error out"=w400:errorcluster)
          }
          event "Run Sweep": Value Change {
            n148 = event-data() -> ()  [unwired: 1 in, 1 out]
            n149 = local read "Power Scaling.0"() -> (w409:dbl)
            n150 = local read "Eb/N0 (dB).0"() -> (w410:dbl)
            n151 = Bundle("Eb/N0 (dB).0"=w410, "Power Scaling.0"=w409) -> (w408:T17)  [unwired: 1 in]
            n152 = Bundle By Name(cluster=w412, "Inc"=FALSE, "Sweeping Type"="Sweeping Type.0", "Sweeping Start Point"=w408, "Sweeping Current Point"=w408) -> (w414:T16)
            n153 = property on="Generation Mode.0" class="CmbBox"(error in=w404, "Val(Sgnl)"="Pulsed BPSK Modulator" ("Value (Signaling)")) -> (error out=w405:errorcluster)  [unwired: 1 in, 1 out]
            n154 = Generate User Event(user event=w419, event data cluster=w414, error in=w405) -> (error out=w418:errorcluster)  [unwired: 1 in, 1 out]
            n155 = Generate User Event(user event=w417, event data cluster="", error in=w418) -> (error out=w413:errorcluster)  [unwired: 1 in, 1 out]
          }
          event User Event {
            n156 = event-data() -> ("Sweeping Type"=w434:enum16{"Eb/N0", "Power"}, "Sweeping Start Point"=w433:cluster{"Eb/N0":dbl, "Power Scaling":dbl}, "Sweeping Current Point"=w432:cluster{"Eb/N0":dbl, "Power Scaling":dbl}, "Inc"=w431:bool)  [unwired: 1 in]
            n157 = case shown="\"Eb/N0\"" w434 {
              selector: w434 -> [w445 w469]
              tunnel: [w455 w476] -> w429
              tunnel: [w453 w474] -> w430
              tunnel: w435 -> [w451 w473]
              tunnel: w433 -> [w443 w468]
              tunnel: w432 -> [w448 w467]
              tunnel: w431 -> [w447 w472]
              frame "Eb/N0" {
                n158 = Unbundle(w448) -> ("Eb/N0"=w449:dbl)  [unwired: 1 out]
                n159 = case shown="False" w447 {
                  tunnel: w449 -> [w460 w463]
                  tunnel: 0.06 ("x") -> [w459 w462]
                  tunnel: [w458 w461] -> w452
                  frame False {
                    n160 = Subtract(x=w460, y=w459) -> (x-y=w458:dbl)
                  }
                  frame True {
                    n161 = Add(x=w463, y=w462) -> (x+y=w461:dbl)
                  }
                }
                n162 = Bundle(cluster=w448, "Eb/N0"=w452) -> (w444:cluster{"Eb/N0":dbl, "Power Scaling":dbl})  [unwired: 1 in]
                n163 = Unbundle(w443) -> ("Eb/N0"=w450:dbl)  [unwired: 1 out]
                n164 = Less Or Equal To 0?(x=w452) -> (x <= 0?=w456:bool)
                n165 = Greater Or Equal?(x=w452, y=w450) -> (x >= y?=w454:bool)
                n166 = Or(x=w447, y=w456) -> (x .or. y?=w446:bool)
                n167 = And(x=w454, y=w447) -> (x .and. y?=w453:bool)
                n168 = Bundle(cluster=w451, "Inc"=w446, "Sweeping Type"=w445, "Sweeping Start Point"=w443, "Sweeping Current Point"=w444) -> (w455:T16)
              }
              frame "Power" {
                n169 = Unbundle(w467) -> ("Power Scaling"=w464:dbl)  [unwired: 1 out]
                n170 = Unbundle(w468) -> ("Power Scaling"=w465:dbl)  [unwired: 1 out]
                n171 = case shown="True" w472 {
                  tunnel: w464 -> [w481 w484]
                  tunnel: 0.002 ("x") -> [w480 w483]
                  tunnel: [w479 w482] -> w471
                  frame False {
                    n172 = Subtract(x=w481, y=w480) -> (x-y=w479:dbl)
                  }
                  frame True {
                    n173 = Add(x=w484, y=w483) -> (x+y=w482:dbl)
                  }
                }
                n174 = Bundle(cluster=w467, "Power Scaling"=w471) -> (w466:cluster{"Eb/N0":dbl, "Power Scaling":dbl})  [unwired: 1 in]
                n175 = Less Or Equal To 0?(x=w471) -> (x <= 0?=w477:bool)
                n176 = Greater Or Equal?(x=w471, y=w465) -> (x >= y?=w475:bool)
                n177 = Or(x=w472, y=w477) -> (x .or. y?=w470:bool)
                n178 = And(x=w475, y=w472) -> (x .and. y?=w474:bool)
                n179 = Bundle(cluster=w473, "Inc"=w470, "Sweeping Type"=w469, "Sweeping Start Point"=w468, "Sweeping Current Point"=w466) -> (w476:T16)
              }
            }
            n180 = Unbundle(w429) -> ("Sweeping Start Point"=w428:cluster{"Eb/N0":dbl, "Power Scaling":dbl}, "Sweeping Current Point"=w427:cluster{"Eb/N0":dbl, "Power Scaling":dbl})  [unwired: 2 out]
            n181 = Select(t=w428, s=w430, f=w427) -> (s? t:f=w426:cluster{"Eb/N0":dbl, "Power Scaling":dbl})
            n182 = Unbundle(w426) -> ("Eb/N0"=w425:dbl, "Power Scaling"=w424:dbl)
            n183 = property on="Eb/N0 (dB).0" class="DigNum (strict)"(error in=w437, "Val(Sgnl)"=w425) -> (error out=w441:errorcluster)  [unwired: 1 in, 1 out]
            n184 = property on="Power Scaling.0" class="DigNum (strict)"(error in=w441, "Val(Sgnl)"=w424) -> (error out=w436:errorcluster)  [unwired: 1 in, 1 out]
            n185 = case shown="False" w430 {
              tunnel: w440 -> [w491 _]
              tunnel: w436 -> [w490 w492]
              tunnel: w429 -> [w486 _]
              tunnel: [w488 w492] -> w439
              tunnel: w438 -> [w487 _]
              frame False {
                n186 = Generate User Event(user event=w491, event data cluster=w486, error in=w490) -> (error out=w489:errorcluster)  [unwired: 1 in, 1 out]
                n187 = Generate User Event(user event=w487, event data cluster="", error in=w489) -> (error out=w488:errorcluster)  [unwired: 1 in, 1 out]
              }
              frame True {
              }
            }
          }
          event "Eb/N0 (dB).0": Value Change {
            n188 = event-data() -> ("NewVal"=w506:dbl)  [unwired: 1 in]
            n189 = call "HOST Configure AWGN (BPSK).vi"("E0/Nb"=w506) -> ("output data type"=w496:T12, "noise std deviation\n(unity signal power)"=w497:dbl, "seed"=w498:fxp<+,25,25>)  [unwired: 8 in]
            n190 = xnode "Read/Write Control"("FPGA VI Reference In"=w493, "error in"=w502) -> ("FPGA VI Reference Out"=w501:T6, "error out"=w500:errorcluster, "modulator configurations.0"=w499:T10)
            n191 = Bundle By Name(cluster=w499, "AWGN Seed"=w498, "AWGN scaling"=w497, "output type selection"=w496) -> (w495:T10)
            n192 = property on="Generation Mode.0" class="CmbBox"("Val(Sgnl)"="Pulsed BPSK Modulator" ("Value (Signaling)")) -> ()  [unwired: 2 in, 2 out]
            n193 = xnode "Read/Write Control"("FPGA VI Reference In"=w501, "error in"=w500, "modulator configurations.0"=w495) -> ("FPGA VI Reference Out"=w504:T6, "error out"=w505:errorcluster)
          }
          event "Power Scaling.0": Value Change {
            n194 = event-data() -> ("NewVal"=w509:dbl)  [unwired: 1 in]
            n195 = xnode "Read/Write Control"("FPGA VI Reference In"=w508, "error in"=w516) -> ("FPGA VI Reference Out"=w514:T6, "error out"=w513:errorcluster, "modulator configurations.0"=w507:T10)
            n196 = Bundle By Name(cluster=w507, "power scaling"=w509) -> (w510:T10)
            n197 = xnode "Read/Write Control"("FPGA VI Reference In"=w514, "error in"=w513, "modulator configurations.0"=w510) -> ("FPGA VI Reference Out"=w511:T6, "error out"=w512:errorcluster)
          }
          event Panel Close? {
            w519 = TRUE
            n198 = event-data() -> ()  [unwired: 1 in, 1 out]
            n199 = event-data("Discard?"=w519) -> ()  [unwired: 1 in, 1 out]
          }
          event "stop": Value Change {
            n200 = event-data() -> ()  [unwired: 1 in, 1 out]
          }
        }
        n201 = local write "Status"("Generating Signal" ("Status")) -> ()
        n202 = Or(x=w271, y=w275) -> (x .or. y?=w272:bool)
      }
      n203 = Destroy User Event(user event=w247, error in=w250) -> (error out=w249:errorcluster)
      n204 = Destroy User Event(user event=w246, error in=w249) -> (error out=w248:errorcluster)
      n205 = Unregister For Events(event registration refnum=w251, error in=w248) -> (error out=w238:errorcluster)
      n206 = Select(t="Error Generating", s=w250, f="Stopped") -> (s? t:f=w255:string)
    }
    frame Error {
    }
  }
  "Status" <- w64
  n207 = local read "Coprocessor Device Name"() -> (w49:T4)
  n208 = call-poly <vilib>:"Close References.vi"("device name"=w49, "error in"=w50, "session in"=w51) -> ("error out"=w13:errorcluster, "session out"=w14:T7)  [unwired: 7 in]
  n209 = call <vilib>:"Release Session.vi"("error in"=w13, "session in"=w14) -> ("error out"=w57:errorcluster)  [unwired: 8 in, 1 out]
  n210 = xnode "Close FPGA VI Reference"("FPGA VI Reference In"=w59) -> ("error out"=w58:errorcluster)  [unwired: 1 in]
  n211 = Merge Errors(w57, w58) -> (w53:errorcluster)
  n212 = call <vilib>:"Simple Error Handler.vi"("error in (no error)"=w53) -> ()  [unwired: 4 in, 5 out]
